vi "REPORT.BIN TO STRING ACTIVE TEST.vi"(2 "realizar test?":bool, 7 "OK o Fault":string) -> (8 "(OK, Fault) (No data)":string)   [LabVIEW 2019]
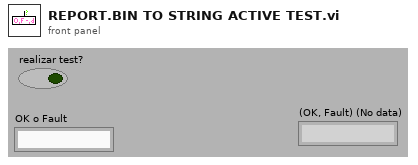
[diagram p1: front panel]
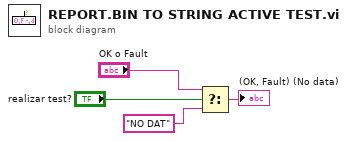
[diagram p0: block diagram]
diagram:
  n1 = Select(t="OK o Fault", s="realizar test?", f="NO DAT") -> (s? t:f=→"(OK, Fault) (No data)":string)
